vi "UHR-Fleezers Control (host) -TL - oscillation.vi"(0 "Tab Control":T5(tab)) -> ()   [LabVIEW 2013] (continued)
  n76 = xnode "Read/Write Control"("FPGA VI Reference In"=w122, "error in"=w142, "ai count"="AI Count (ticks)", "Interlace ON/OFF"=w107, "Number Interlace Cycles"=w106, "AI1 Sets to FIFO"=w235, "FB On/Off Set 1"=w234, "FB On/Off Set 2"=w233, "Interlace Off Parameters"=w105, "FB Setpoint Set 1"=w225, "FB Setpoint Set 2"=w224, "FB Gains Set 1"=w222, "FB Gains Set 2"=w221, "FB output range 1"=w124, "FB output range 2"=w124, "Cycles per step"=w206, "Scan BD"=w218, "Number of scans"=w202, "Scan steps"=w207, "Scan freq.  increment"=w208, "AO1"=w190, "AO2"=w189, "Scan freq.  increment (MCL)"=w183, "Scan steps (MCL)"=w182, "Cycles per step (MCL)"=w181, "Number of scans (MCL)"=w180, "MCL count"=w104, "Cont. Scan (MCL)"=w179, "MCL Scan Axis"=w173, "1D or 2D Scan?"=w125, "N of AI1 Int Acq Sets"=w164, "Freq or Amp switch first"="Freq or Amp switch first", "Freq switch delay"="Freq switch delay", "Amp switch delay"="Amp switch delay", "Swap F1 and F2"="Swap F1 and F2", "APD Acq Rate Count"=w130, "APD to FIFO"=FALSE, "APD Gate Operating Mode"="APD Gate", "APD Gate ON Count"="APD Gate ON Count", "APD Gate OFF Count"="APD Gate OFF Count", "Invert APD Gate"="Invert APD Gate", "DIO count 1 (ticks)"="DIO count 1 (ticks)", "DIO count 2 (ticks)"="DIO count 2 (ticks)", "DIO count 3 (ticks)"="DIO count 3 (ticks)", "APD 1 AO scale factor"="APD 1 AO Mult.", "APD 2 AO scale factor"="APD 2 AO Mult.") -> ("FPGA VI Reference Out"=w99:T19, "error out"=w101:errorcluster)  [unwired: 1 in]
  n77 = local read "Green Laser ON/Interlacing"() -> (w102:bool)
  n78 = local read "Green laser mode"() -> (w103:enum32{"Laser ON", "Laser OFF", "Interlace"})
  n79 = local read "GI Frequency, OFF count"() -> (w95:u32)
  n80 = local read "GI Frequency, ON count"() -> (w94:u32)
  n81 = Multiply(x="Current When FB OFF (%)", y=655.35) -> (x*y=w85:dbl)
  n82 = local read "Green FB Count"() -> (w93:u32)
  n83 = Multiply(x="Green FB Setpoint (mV)", y=3.2767) -> (x*y=w82:dbl)
  n84 = To Unsigned Word Integer(number=w85) -> (unsigned 16bit integer=w83:u16)
  n85 = local read "Invert GI"() -> (w97:bool)
  n86 = To Word Integer(number=w82) -> (16bit integer=w80:i16)
  n87 = case shown="True" w102 {
    tunnel: w103 -> [_ w255]
    tunnel: [enum32{"Laser ON", "Laser OFF", "Interlace"}."Laser OFF" ("Green laser mode") w255] -> w96
    frame False {
    }
    frame True {
    }
  }
  n88 = local read "Trap Pos. AI1 X Pre-scale"() -> (w51:u16)
  n89 = local read "Trap Pos FB Monitor\nT1 or T2"() -> (w58:bool)
  n90 = local read "Trap Pos FB Int Count"() -> (w46:u16)
  n91 = local read "Trap Pos FB Negate Action"() -> (w57:bool)
  n92 = local read "Trap Pos. FB Offset Factor"() -> (w56:i64)
  n93 = local read "Trap Pos. FB Mult Factor"() -> (w55:i64)
  n94 = local read "Trap Pos. FB Gains"() -> (w53:T11)
  n95 = local read "Trap Pos. FB Range"() -> (w54:T12)
  n96 = xnode "Read/Write Control"("FPGA VI Reference In"=w99, "error in"=w101, "Green interlace ON count 2"=w94, "Green interlace OFF count 2"=w95, "Invert GI 2"=w97, "Operating Mode 2"=w96, "Green FB Gains"="Green FB Gains", "Green FB Setpoint"=w80, "Green FB On/Off"="Green FB On/Off", "Current Out"=w83, "Green int current ON count adj"="Green int current ON count adj", "Green FB Count"=w93, "Operating Mode"=w96, "Green interlace OFF count"=w95, "Green interlace ON count"=w94, "Invert GI"=w97, "Trap Pos FB Monitor T1 or T2"=w58, "Trap Pos FB Negate Action"=w57, "Trap Pos. FB Offset Factor"=w56, "Trap Pos. FB Mult Factor"=w55, "Trap Pos. FB Range"=w54, "Trap Pos. FB Gains"=w53, "Force feedback"=FALSE, "AI1 X Scale"=w51, "Trap Pos to FIFO"=TRUE, "Trap Pos FB Int Count"=w46) -> ("FPGA VI Reference Out"=w98:T19, "error out"=w100:errorcluster)
  n97 = xnode "Invoke Method"("FPGA VI Reference In"=w98, "error in"=w100, "Requested Depth"="Trap AI FIFO Depth") -> ("FPGA VI Reference Out"=w61:T19, "error out"=w60:errorcluster)  [unwired: 1 out]
  n98 = xnode "Invoke Method"("FPGA VI Reference In"=w61, "error in"=w60, "Requested Depth"="Trap Position FIFO Depth") -> ("FPGA VI Reference Out"=w48:T19, "error out"=w47:errorcluster)  [unwired: 1 out]
  n99 = flat-sequence {
    tunnel: w123 -> [w260]
    tunnel: [w260] -> w122
    tunnel: [w259] -> w121
    tunnel: [w258] -> w120
    tunnel: [w256] -> w118
    tunnel: [w257] -> w119
    frame #0 {
      w257 = T16 {"Minimum"=50.0, "Maximum"=100.0, "Increment"=1.0} ("Min Max Inc")
      w256 = T16 {"Minimum"=0.0, "Maximum"=75.0, "Increment"=1.0} ("Data Entry Limits")
      w259 = T16 {"Minimum"=50.0, "Maximum"=100.0, "Increment"=1.0} ("Min Max Inc")
      w258 = T16 {"Minimum"=0.0, "Maximum"=75.0, "Increment"=1.0} ("Data Entry Limits")
      n100 = property on="BD 2 Frequency 1 (MHz)" class="DigNum (strict)"("Data Range"=w257) -> ()  [unwired: 2 in, 2 out]
      n101 = property on="BD 2 Frequency 3 (MHz)" class="DigNum (strict)"("Data Range"=w257) -> ()  [unwired: 2 in, 2 out]
      n102 = property on="BD 2 Frequency 2 (MHz)" class="DigNum (strict)"("Data Range"=w257) -> ()  [unwired: 2 in, 2 out]
      n103 = property on="BD 1 Frequency 1 (MHz)" class="DigNum (strict)"("Data Range"=w259) -> ()  [unwired: 2 in, 2 out]
      n104 = property on="BD 1 Frequency 2 (MHz)" class="DigNum (strict)"("Data Range"=w259) -> ()  [unwired: 2 in, 2 out]
      n105 = property on="BD 1 Frequency 3 (MHz)" class="DigNum (strict)"("Data Range"=w259) -> ()  [unwired: 2 in, 2 out]
      n106 = property on="BD 2 Amplitude 1 (%)" class="DigNum (strict)"("Data Range"=w256) -> ()  [unwired: 2 in, 2 out]
      n107 = property on="BD 2 Amplitude 2 (%)" class="DigNum (strict)"("Data Range"=w256) -> ()  [unwired: 2 in, 2 out]
      n108 = property on="BD 2 Amplitude 3 (%)" class="DigNum (strict)"("Data Range"=w256) -> ()  [unwired: 2 in, 2 out]
      n109 = property on="BD 1 Amplitude 3 (%)" class="DigNum (strict)"("Data Range"=w258) -> ()  [unwired: 2 in, 2 out]
      n110 = property on="BD 1 Amplitude 2 (%)" class="DigNum (strict)"("Data Range"=w258) -> ()  [unwired: 2 in, 2 out]
      n111 = property on="BD 1 Amplitude 1 (%)" class="DigNum (strict)"("Data Range"=w258) -> ()  [unwired: 2 in, 2 out]
      "X RF Frequency Limits (MHz)" <- w259
      "X RF Amplitude Limits (%)" <- w258
      "Y RF Amplitude Limits (%)" <- w256
      "Y RF Frequency Limits (MHz)" <- w257
    }
  }
  n112 = xnode "Invoke Method"("FPGA VI Reference In"=w48, "error in"=w47) -> ("FPGA VI Reference Out"=w27:T19, "error out"=w26:errorcluster)  [unwired: 1 in]
  n113 = flat-sequence "Initial FPGA Loop Relative Phase Adjustment" {
    tunnel: "Initial Phase Adjustment (APD 2 Gate)" -> [w262]
    tunnel: "Initial Phase Adjustment (GI) 2" -> [w263]
    tunnel: "Initial Phase Adj. (MCL)" -> [w264]
    tunnel: w26 -> [w265]
    tunnel: w27 -> [w266]
    tunnel: "Initial Phase Adjustment (GI)" -> [w267]
    tunnel: "Initial Phase Adjustment (AI1)" -> [w268]
    tunnel: [w268] -> w35
    tunnel: [w267] -> w34
    tunnel: [w266] -> w33
    tunnel: [w265] -> w32
    tunnel: [w264] -> w31
    tunnel: [w263] -> w30
    tunnel: [w262] -> w29
    tunnel: [w280] -> w148
    tunnel: [w274] -> w146
    tunnel: "Initial Phase Adjustment (APD Acq)" -> [w273]
    tunnel: "Initial Phase Adjustment (APD 1 Gate)" -> [w272]
    tunnel: "Initial Phase Adjustment (Green FB)" -> [w271]
    tunnel: w35 -> [w279]
    tunnel: w34 -> [w278]
    tunnel: w33 -> [w277]
    tunnel: w32 -> [w276]
    tunnel: w31 -> [w275]
    tunnel: w30 -> [w270]
    tunnel: w29 -> [w269]
    tunnel: w148 -> [w282]
    tunnel: [w283] -> w147
    tunnel: w146 -> [w283]
    tunnel: [w282] -> w145
    tunnel: w147 -> [w286]
    tunnel: w145 -> [w285]
    tunnel: [w288] -> w144
    tunnel: [w287] -> w143
    tunnel: [w290] -> w25
    tunnel: [w291] -> w28
    tunnel: w144 -> [w291]
    tunnel: w143 -> [w290]
    frame #0 {
      n114 = Wait (ms)(milliseconds to wait=u32 1000) -> ()  [unwired: 1 out]
    }
    frame #1 {
      n115 = xnode "Read/Write Control"("FPGA VI Reference In"=w277, "error in"=w276, "Phase count adjustment"=w279, "Phase count adjustment (GI)"=w278, "Phase count adjustment (MCL)"=w275, "Phase Count Adjustment (APD Acq)"=w273, "Phase count adjustment (APD 1 Gate)"=w272, "Phase count adjustment (APD 2 Gate)"=w269, "Phase count adjustment (Green FB)"=w271, "Phase count adjustment (GI) 2"=w270) -> ("FPGA VI Reference Out"=w274:T19, "error out"=w280:errorcluster)
    }
    frame #2 {
      n116 = Wait (ms)(milliseconds to wait=u32 1000) -> ()  [unwired: 1 out]
    }
    frame #3 {
      w284 = TRUE
      n117 = xnode "Read/Write Control"("FPGA VI Reference In"=w286, "error in"=w285, "+ phase"=w284, "+ phase (GI)"=w284, "+ phase (MCL)"=w284, "+ phase (APD Acq)"=w284, "+ phase (APD 1 Gate)"=w284, "+ phase (APD 2 Gate)"=w284, "+ phase (Green FB)"=w284, "+ phase (GI) 2"=w284) -> ("FPGA VI Reference Out"=w287:T19, "error out"=w288:errorcluster)
    }
    frame #4 {
      n118 = Wait (ms)(milliseconds to wait=u32 1000) -> ()  [unwired: 1 out]
    }
  }
  n119 = local read "Phase adj. (Green FB)"() -> (w116:i16)
  n120 = local read "Phase adj. (GI) 2"() -> (w86:i16)
  n121 = local read "Phase adjust (MCL)"() -> (w174:i16)
  n122 = local read "Phase adj. (AI1)"() -> (w176:i16)
  n123 = local read "Phase adj. (GI)"() -> (w175:i16)
  n124 = xnode "Read/Write Control"("FPGA VI Reference In"=w25, "error in"=w28, "Phase count adjustment"=w176, "Phase count adjustment (GI)"=w175, "Phase count adjustment (MCL)"=w174, "Phase Count Adjustment (APD Acq)"="Phase Adj. (APD Acq)", "Phase count adjustment (APD 1 Gate)"="Phase Adj. (APD 1 Gate)", "Phase count adjustment (APD 2 Gate)"="Phase Adj. (APD 2 Gate)", "Phase count adjustment (Green FB)"=w116, "Phase count adjustment (GI) 2"=w86) -> ("FPGA VI Reference Out"=w24:T19, "error out"=w23:errorcluster)
  n125 = call "Initialize RF boards - interlace 3.vi"("error in"=w23, "FPGA VI Reference In"=w24) -> ("FPGA VI Reference Out"=w153:T19)  [unwired: 1 out]
  n126 = call "set RF board frequency - interlace.vi"("Board 2 Frequency Limits"=w119, "Board 1 Frequency Limits"=w121, "FPGA VI Reference In"=w153, "Board 2 Frequency 3 (MHz)"="BD 2 Frequency 3 (MHz)", "Board 1 Frequency 3 (MHz)"="BD 1 Frequency 3 (MHz)", "Board 2 Frequency 2 (MHz)"="BD 2 Frequency 2 (MHz)", "Board 2 Frequency 1 (MHz)"="BD 2 Frequency 1 (MHz)", "Board 1 Frequency 2 (MHz)"="BD 1 Frequency 2 (MHz)", "Board 1 Frequency 1  (MHz)"="BD 1 Frequency 1 (MHz)") -> ("error out"=w246:errorcluster, "FPGA VI Reference Out"=w247:T19)  [unwired: 1 in]
  n127 = call "set RF board amplitude - interlace.vi"("Board 2 Amplitude Limits"=w118, "Board 1 Amplitude Limits"=w120, "error in"=w246, "FPGA VI Reference In"=w247, "Board 2 Amplitude 3 (%)"="BD 2 Amplitude 3 (%)", "Board 1 Amplitude 3 (%)"="BD 1 Amplitude 3 (%)", "Board 2 Amplitude 2 (%)"="BD 2 Amplitude 2 (%)", "Board 2 Amplitude 1 (%)"="BD 2 Amplitude 1 (%)", "Board 1 Amplitude 2 (%)"="BD 1 Amplitude 2 (%)", "Board 1 Amplitude 1 (%)"="BD 1 Amplitude 1 (%)") -> ("error out"=w21:errorcluster, "FPGA VI Reference Out"=w22:T19)
  n128 = flat-sequence {
    tunnel: w22 -> [w300]
    tunnel: w21 -> [w299]
    tunnel: [w298] -> w239
    tunnel: [w297] -> w238
    tunnel: [w304] -> w237
    tunnel: w239 -> [w304]
    tunnel: [w303] -> w236
    tunnel: w238 -> [w303]
    tunnel: w237 -> [w313]
    tunnel: w236 -> [w312]
    tunnel: [w311] -> w17
    tunnel: [w306] -> w16
    tunnel: [w316] -> w44
    tunnel: [w320] -> w2
    tunnel: w17 -> [w320]
    tunnel: w16 -> [w315]
    frame #0 {
      n129 = local read "Trap 1 (ON/OFF)"() -> (w292:bool)
      n130 = xnode "Read/Write Control"("FPGA VI Reference In"=w300, "error in"=w299, "Direct RF Box  Communication"=FALSE) -> ("FPGA VI Reference Out"=w298:T19, "error out"=w297:errorcluster)
      n131 = local write "Saving..."(FALSE ("Saving Data")) -> ()
      n132 = local write "Stop All"(FALSE ("Stop All")) -> ()
      n133 = local write "Index"(1.0 ("Index")) -> ()
      n134 = property on="Trap 1 ON" class="Bool (strict)"("Value"=w292) -> ()  [unwired: 2 in, 2 out]
      "Manipulating Trap" <- FALSE ("Manipulating Trap")
    }
    frame #1 {
      n135 = local read "Trap 2 (ON/OFF)"() -> (w302:bool)
      n136 = Wait (ms)(milliseconds to wait=u32 50) -> ()  [unwired: 1 out]
      n137 = property on="Trap 2 ON" class="Bool (strict)"("Val(Sgnl)"=w302) -> ()  [unwired: 2 in, 2 out]
    }
    frame #2 {
      n138 = local read "Scan Range (nm)"() -> (w307:dbl)
      n139 = xnode "Read/Write Control"("FPGA VI Reference In"=w313, "error in"=w312, "FPGA Controls  RF Box"=TRUE ("Direct RF Box  Communication")) -> ("FPGA VI Reference Out"=w311:T19, "error out"=w306:errorcluster)
      n140 = call "Update messages.vi"("Message to add"="UHR-Fleezers ready.", "Old message string"="") -> ("New message string"=w310:string)
      n141 = local write "Messages"(w310) -> ()
      n142 = property on="Scan Range (nm)" class="DigNum (strict)"("Val(Sgnl)"=w307) -> ()  [unwired: 2 in, 2 out]
    }
    frame #3 {
      n143 = call "hamilton_controller.vi"("error in"=w315, "action"=T20."CONNECT") -> ("error out"=w317:errorcluster)  [unwired: 9 in]
      n144 = call "hamilton_controller.vi"("error in"=w317, "action"=T20."INITIALIZE VALVES") -> ("error out"=w316:errorcluster)  [unwired: 9 in]
    }
  }
  n145 = Subtract(x="BD 1 Frequency 1 (MHz)", y="BD 1 Frequency 2 (MHz)") -> (x-y=w163:dbl)
  n146 = Subtract(x="BD 2 Frequency 1 (MHz)", y="BD 2 Frequency 2 (MHz)") -> (x-y=w162:dbl)
  n147 = Square(x=w162) -> (x^2=w160:dbl)
  n148 = Square(x=w163) -> (x^2=w161:dbl)
  n149 = Add(x=w161, y=w160) -> (x+y=w159:dbl)
  n150 = Square Root(x=w159) -> (sqrt(x)=w158:dbl)
  n151 = local write "Trap Delta (MHz)"(w158) -> ()
  n152 = call "IMAQ Create"("Image Name"="APD 1 Image", "Image Type"=w67) -> ("New Image"=w66:T3)  [unwired: 3 in, 1 out]
  n153 = call "IMAQ Create"("Image Name"="APD 2 Image", "Image Type"=w67) -> ("New Image"=w65:T3)  [unwired: 3 in, 1 out]
  n154 = call "IMAQ Create"("Image Name"="Det. X Image", "Image Type"=w67) -> ("New Image"=w64:T3)  [unwired: 3 in, 1 out]
  n155 = call "IMAQ Create"("Image Name"="Det. Y Image", "Image Type"=w67) -> ("New Image"=w63:T3)  [unwired: 3 in, 1 out]
  n156 = Bundle("New Image"=w66, "New Image"=w65, "New Image"=w64, "New Image"=w63) -> (w62:T21)  [unwired: 1 in]
  n157 = Current VI's Path() -> (path=w6:path)
  n158 = Concatenate Strings("N.D.", "\r\n") -> (w10:string)
  n159 = Strip Path(path=w6) -> (stripped path=w7:path)  [unwired: 1 out]
  n160 = Initialize Array(w10, 4, 3) -> (w13:string[][])
  n161 = Build Path(base path=w7, name or relative path="Locations.txt") -> (appended path=→"Location path":path)
  n162 = local write "Location Matrix"(w13) -> ()
  n163 = while {
    stop <- w321 stop-if-true
    n164 = event shown="[1] \"Goto Top (F6)\": Value Change" {
      selector: _ -> [_ _ _ _ _ _ _]
      dyn-events: _ -> [_ _ _ _ _ _ _]
      timeout: 10 -> [_ _ _ _ _ _ _]
      tunnel: [FALSE _ _ _ _ _ _] -> w321
      event Timeout {
        # "Change the trajectory mode to Jog"
        # "Query and display stage positions"
        # "Setting ESP300 left and right limits for Z-axis, input in mm"
        # "Display Selected Location"
        n165 = event-data() -> ()  [unwired: 1 in, 2 out]
        n166 = local read "Capture Locations"() -> (w346:i32)
        n167 = local read "Location Matrix"() -> (w347:string[][])
        n168 = Concatenate Strings("1TP;\n2TP;\n3TP;\n1MD?;\n2MD?;\n3MD?" ("Substring"), "\r") -> (w330:string)
        n169 = local read "ESP Port"() -> (w333:refnum<visa-resource-name>)
        n170 = Index Array(array=w347, index (row)=w346) -> (element=w345:string[])  [unwired: 1 in]
        n171 = local read "ESP Port"() -> (w342:refnum<visa-resource-name>)
        n172 = VISA Write(VISA resource name=w333, write buffer=w330, error in (no error)="error in") -> (VISA resource name out=w331:refnum<visa-resource-name>, error out=w329:errorcluster)  [unwired: 1 out]
        n173 = Concatenate Strings("3SL" ("Substring"), "ESP ZL-Limit", ";3SR", "ESP ZR-Limit", "\r") -> (w341:string)
        n174 = Array To Cluster(array=w345) -> (cluster=w344:T22)
        n175 = case shown="True" TRUE ("Case Constant\n(See Context Help)") {
          tunnel: w331 -> [_ w385]
          tunnel: w329 -> [w366 w384]
          tunnel: [w366 w368] -> w335
          frame False {
          }
          frame True {
            w378 = u16 10 items=["1.0"=10, "1.5"=15, "2.0"=20] ("Serial Settings:Stop Bits")
            w379 = u16 0 items=["None", "Odd", "Even", "Mark", "Space"] ("Serial Settings:Parity")
            n176 = property class="Instr"(reference=w385, error in=w384, "Baud"=u32 921600 ("Serial Settings:Baud Rate"), "Data Bits"=u16 8 ("Serial Settings:Data Bits"), "Parity"=w379, "Stop Bits"=w378) -> (reference out=w383:refnum<visa-resource-name>, error out=w382:errorcluster, "Bytes at Port"=w367:u32)
            n177 = Wait (ms)(milliseconds to wait=u32 10) -> ()  [unwired: 1 out]
            n178 = VISA Read(VISA resource name=w383, byte count=w367, error in (no error)=w382) -> (VISA resource name out=w391:refnum<visa-resource-name>, read buffer=→"X Pos":string, error out=w392:errorcluster)  [unwired: 1 out]
            n179 = VISA Read(VISA resource name=w391, byte count=w367, error in (no error)=w392) -> (VISA resource name out=w389:refnum<visa-resource-name>, read buffer=→"Y Pos":string, error out=w390:errorcluster)  [unwired: 1 out]
            n180 = VISA Read(VISA resource name=w389, byte count=w367, error in (no error)=w390) -> (VISA resource name out=w377:refnum<visa-resource-name>, read buffer=→"Z Pos Pos":string, error out=w376:errorcluster)  [unwired: 1 out]
            n181 = VISA Read(VISA resource name=w377, byte count=w367, error in (no error)=w376) -> (VISA resource name out=w373:refnum<visa-resource-name>, read buffer=→"X Motion":string, error out=w374:errorcluster)  [unwired: 1 out]
            n182 = VISA Read(VISA resource name=w373, byte count=w367, error in (no error)=w374) -> (VISA resource name out=w372:refnum<visa-resource-name>, read buffer=→"Y Motion":string, error out=w370:errorcluster)  [unwired: 1 out]
            n183 = VISA Read(VISA resource name=w372, byte count=w367, error in (no error)=w370) -> (read buffer=→"Z motion":string, error out=w368:errorcluster)  [unwired: 2 out]
          }
        }
        "error out" <- w335
        n184 = VISA Write(VISA resource name=w342, write buffer=w341) -> ()  [unwired: 1 in, 3 out]
        n185 = local write item#485(w344) -> ()
        n186 = disable-structure shown="Disabled" {
          frame Disabled {
            # "Change Low Jog Velocity"
            # "Change High Jog Velocity"
            n187 = Concatenate Strings("1JH" ("Substring"), "Axis 1", "2JH" ("Substring"), "Axis 2", "3JH" ("Substring"), "Axis 3", "\r") -> (w365:string)
            n188 = local read "ESP Port"() -> (w364:refnum<visa-resource-name>)
            n189 = VISA Write(VISA resource name=w364, write buffer=w365) -> ()  [unwired: 1 in, 3 out]
            n190 = Concatenate Strings("1JW" ("Substring"), "Axis 1", "2JW" ("Substring"), "Axis 2", "3JW" ("Substring"), "Axis 3", "\r") -> (w356:string)
            n191 = local read "ESP Port"() -> (w355:refnum<visa-resource-name>)
            n192 = VISA Write(VISA resource name=w355, write buffer=w356) -> ()  [unwired: 1 in, 3 out]
          }
          frame Enabled {
          }
        }
        n193 = local read "ESP Port"() -> (w323:refnum<visa-resource-name>)
        n194 = Concatenate Strings("1TJ3;\n2TJ3;\n3TJ3" ("Substring"), "\r") -> (w324:string)
        n195 = VISA Write(VISA resource name=w323, write buffer=w324) -> ()  [unwired: 1 in, 3 out]
      }
      event "Goto Top (F6)": Value Change {
        n196 = event-data() -> ()  [unwired: 1 in, 5 out]
        n197 = stacked-sequence {
          frame #0 {
            # "stop motions of all axes before going to avoid reversing of direction"
            n198 = local read "ESP Port"() -> (w397:refnum<visa-resource-name>)
            n199 = Concatenate Strings("ST" ("Substring"), "\r") -> (w394:string)
            n200 = VISA Write(VISA resource name=w397, write buffer=w394) -> ()  [unwired: 1 in, 3 out]
          }
          frame #1 {
            n201 = Wait (ms)(milliseconds to wait=u32 50) -> ()  [unwired: 1 out]
          }
          frame #2 {
            # "Change the trajectory mode to Trapezoidal"
            n202 = local read "ESP Port"() -> (w402:refnum<visa-resource-name>)
            n203 = Concatenate Strings("1TJ1;\n2TJ1;\n3TJ1" ("Substring"), "\r") -> (w399:string)
            n204 = VISA Write(VISA resource name=w402, write buffer=w399) -> ()  [unwired: 1 in, 3 out]
          }
          frame #3 {
            # "Go to Top Dispensor"
            n205 = local read "Location Matrix"() -> (w414:string[][])
            n206 = Index Array(array=w414, index (row)=0) -> (element=w410:string[])  [unwired: 1 in]
            n207 = Decimate 1D Array(w410) -> (w408:string[], w406:string[], w404:string[])
            n208 = local read "ESP Port"() -> (w411:refnum<visa-resource-name>)
            n209 = Concatenate Strings("1PA" ("Substring"), w408, "2PA" ("Substring"), w406, "3PA" ("Substring"), w404, "\r") -> (w412:string)
            n210 = VISA Write(VISA resource name=w411, write buffer=w412) -> ()  [unwired: 1 in, 3 out]
          }
          frame #4 {
            n211 = Wait (ms)(milliseconds to wait=u32 100) -> ()  [unwired: 1 out]
          }
          frame #5 {
            # "Change the trajectory mode to Jog"
            n212 = local read "ESP Port"() -> (w419:refnum<visa-resource-name>)
            n213 = Concatenate Strings("1TJ3;\n2TJ3;\n3TJ3" ("Substring"), "\r") -> (w416:string)
            n214 = VISA Write(VISA resource name=w419, write buffer=w416) -> ()  [unwired: 1 in, 3 out]
          }
        }
      }
      event "Goto Exp (F8)": Value Change {
        n215 = event-data() -> ()  [unwired: 1 in, 5 out]
        n216 = stacked-sequence {
          frame #0 {
            # "stop motions of all axes before going to avoid reversing of direction"
            n217 = local read "ESP Port"() -> (w423:refnum<visa-resource-name>)
            n218 = Concatenate Strings("ST" ("Substring"), "\r") -> (w420:string)
            n219 = VISA Write(VISA resource name=w423, write buffer=w420) -> ()  [unwired: 1 in, 3 out]
          }
          frame #1 {
            n220 = Wait (ms)(milliseconds to wait=u32 50) -> ()  [unwired: 1 out]
          }
          frame #2 {
            # "Change the trajectory mode to Trapezoidal"
            n221 = local read "ESP Port"() -> (w428:refnum<visa-resource-name>)
            n222 = Concatenate Strings("1TJ1;\n2TJ1;\n3TJ1" ("Substring"), "\r") -> (w425:string)
            n223 = VISA Write(VISA resource name=w428, write buffer=w425) -> ()  [unwired: 1 in, 3 out]
          }
          frame #3 {
            # "Go to Experimental"
            n224 = local read "Location Matrix"() -> (w440:string[][])
            n225 = Index Array(array=w440, index (row)=2) -> (element=w436:string[])  [unwired: 1 in]
            n226 = Decimate 1D Array(w436) -> (w434:string[], w432:string[], w430:string[])
            n227 = Concatenate Strings("1PA" ("Substring"), w434, "2PA" ("Substring"), w432, "3PA" ("Substring"), w430, "\r") -> (w438:string)
            n228 = local read "ESP Port"() -> (w437:refnum<visa-resource-name>)
            n229 = VISA Write(VISA resource name=w437, write buffer=w438) -> ()  [unwired: 1 in, 3 out]
          }
          frame #4 {
            n230 = Wait (ms)(milliseconds to wait=u32 200) -> ()  [unwired: 1 out]
          }
          frame #5 {
            # "Change the trajectory mode to Jog"
            n231 = local read "ESP Port"() -> (w442:refnum<visa-resource-name>)
            n232 = Concatenate Strings("1TJ3;\n2TJ3;\n3TJ3" ("Substring"), "\r") -> (w445:string)
            n233 = VISA Write(VISA resource name=w442, write buffer=w445) -> ()  [unwired: 1 in, 3 out]
          }
        }
      }
      event "Goto Bottom (F7)": Value Change {
        n234 = event-data() -> ()  [unwired: 1 in, 5 out]
        n235 = stacked-sequence {
          frame #0 {
            # "stop motions of all axes before going to avoid reversing of direction"
            n236 = local read "ESP Port"() -> (w449:refnum<visa-resource-name>)
            n237 = Concatenate Strings("ST" ("Substring"), "\r") -> (w446:string)
            n238 = VISA Write(VISA resource name=w449, write buffer=w446) -> ()  [unwired: 1 in, 3 out]
          }
          frame #1 {
            n239 = Wait (ms)(milliseconds to wait=u32 50) -> ()  [unwired: 1 out]
          }
          frame #2 {
            # "Change the trajectory mode to Trapezoidal"
            n240 = local read "ESP Port"() -> (w454:refnum<visa-resource-name>)
            n241 = Concatenate Strings("1TJ1;\n2TJ1;\n3TJ1" ("Substring"), "\r") -> (w451:string)
            n242 = VISA Write(VISA resource name=w454, write buffer=w451) -> ()  [unwired: 1 in, 3 out]
          }
          frame #3 {
            # "Go to Bottom Dispensor"
            n243 = local read "Location Matrix"() -> (w466:string[][])
            n244 = Index Array(array=w466, index (row)=1) -> (element=w462:string[])  [unwired: 1 in]
            n245 = Decimate 1D Array(w462) -> (w460:string[], w458:string[], w456:string[])
            n246 = Concatenate Strings("1PA" ("Substring"), w460, "2PA" ("Substring"), w458, "3PA" ("Substring"), w456, "\r") -> (w464:string)
            n247 = local read "ESP Port"() -> (w463:refnum<visa-resource-name>)
